vi "Do Core.vi"(8 "error in (no error)":errorcluster, 9 "Actor in":refnum<class "Actor.lvclass">, 11 "Reply Message":refnum<class "RequestStatus Msg.lvclass">) -> (0 "error out":errorcluster, 1 "Actor out":refnum<class "Actor.lvclass">, 2 "Reply":variant)   [LabVIEW 2016, in "MyBaseActor.lvlib" / "RequestStatus Msg.lvclass"]
doc: "(<B>Filename</B>: Actor Framework.lvlib:Reply Msg.lvclass:Do Core.vi)\n\nDefines what an actor does when it receives <B>Reply Message</B>. This method also defines the <B>Reply</B> that is returned to the actor that sent <B>Reply Message</B>.\n\nBy default, this method does nothing, and <B>Reply</B> is the ancestor Message class. A child class must override this method to define behavior and specify a child of the Message class to return in the <B>Reply</B> output."
uses:
  RequestStatus Msg.lvclass
  <vilib>/ActorFramework/Actor/Actor.lvclass
  MyBaseActor/MyBaseActor.lvclass
  F:/Program Files (x86)/National Instruments/LabVIEW 2016/vi.lib/ActorFramework/Actor/Actor.lvclass
  RequestStatus Msg.lvclass/RequestStatus Msg.ctl
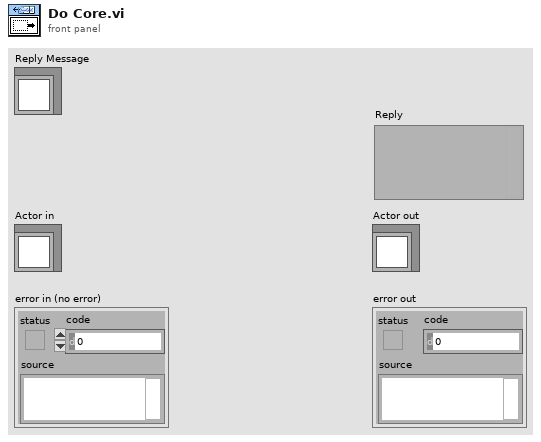
[diagram p1: front panel]
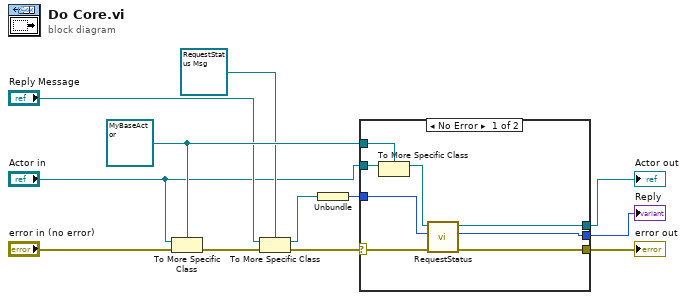
[diagram p0: block diagram]
diagram:
  w11 = refnum<class "MyBaseActor.lvclass"> refnum ("Actor in")
  n1 = To More Specific Class(target class=w11, reference="Actor in", error in="error in (no error)") -> (error out=w2:errorcluster)  [unwired: 1 out]
  n2 = To More Specific Class(target class=refnum<class "RequestStatus Msg.lvclass"> refnum ("RequestStatus Msg"), reference="Reply Message", error in=w2) -> (specific class reference=w8:refnum<class "RequestStatus Msg.lvclass">, error out=w1:errorcluster)
  n3 = Unbundle(w8) -> (w12:i32)
  n4 = case shown="No Error" w1 {
    selector: w1 -> [w18 w22]
    tunnel: [w20 w22] -> w3
    tunnel: [w19 w21] -> w6
    tunnel: "Actor in" -> [w17 w21]
    tunnel: w11 -> [w16 _]
    tunnel: w12 -> [w14 _]
    tunnel: [w13 _] -> w7
    frame No Error {
      n5 = To More Specific Class(target class=w16, reference=w17) -> (specific class reference=w15:refnum<class "MyBaseActor.lvclass">)  [unwired: 1 in, 1 out]
      n6 = call-dynamic "RequestStatus.vi"("error in (no error) 2"=w18, "Data"=w14, "Beta in"=w15) -> ("error out 2"=w20:errorcluster, "x*y"=w13:i32, "Beta out"=w19:refnum<class "MyBaseActor.lvclass">)  [unwired: 6 in]
    }
    frame Error {
      # "If type check fails, pass the original object out again."
    }
  }
  "error out" <- w3
  "Actor out" <- w6
  "Reply" <- w7
